vi "GET Deviation Signal Data.vi"() -> (0 "Deviation Signal Data":dbl[](array[numeric]))   [LabVIEW 2013]
uses:
  Functional Globals/Action.ctl
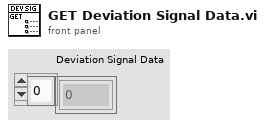
[diagram p1: front panel]
types:
  T1 = typedef "Action.ctl" = enum16{"GET", "PUT", "DELETE"}
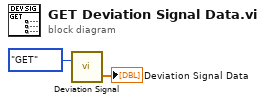
[diagram p0: block diagram]
diagram:
  n1 = call "Deviation Signal.vi"("Action"=Action."GET") -> ("Output"=→"Deviation Signal Data":dbl[])  [unwired: 2 in]
